vi "func_SendERR.vi"(6 "MoreINFO":string, 8 "ERR (String\\Errclust)":variant, 11 "YTESTER测试数据 in":T1) -> (3 "YTESTER测试数据 out":T1)   [LabVIEW 2017]
uses:
  YtCommon.lvlibp/yt`Step TestData.ctl
  YtCommon.lvlibp/yt`Step System Queue.ctl
  YtCommon.lvlibp
panel:
  # "This for Step vi"
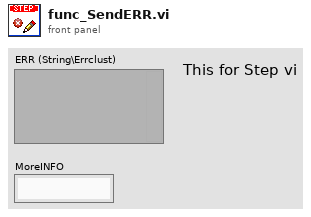
[diagram p1: front panel]
types:
  T1 = typedef "YtCommon.lvlibp/yt`Step TestData.ctl" = cluster{"Socket(From1)":i32, "SN":refnum<notifier>, "StopFlagRef":refnum<notifier>, "YT System Queue":refnum<queue>}
  T2 = typedef "YtCommon.lvlibp/yt`Step System Queue.ctl" = cluster{"Socket(From0)":i32, "Cmd":string, "Data":variant}
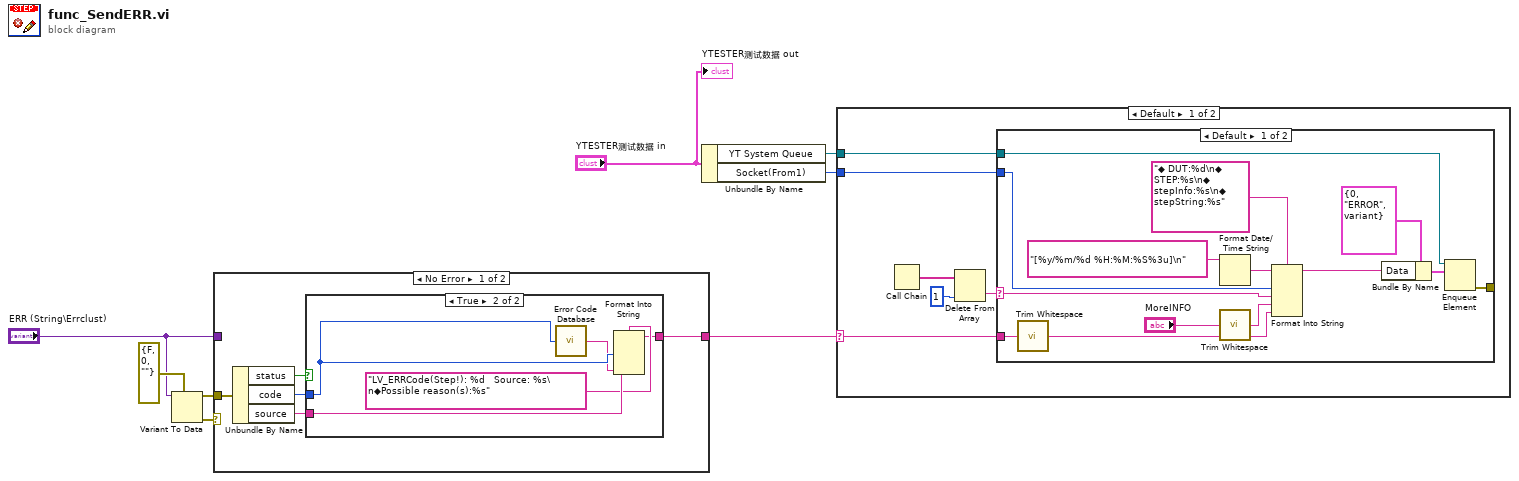
[diagram p0: block diagram]
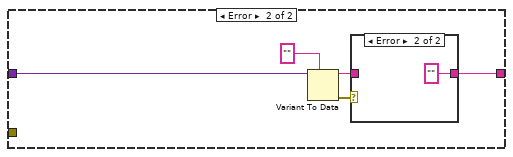
[diagram p5: hidden frame]
diagram:
  n1 = Variant To Data(type=errorcluster {"status"=FALSE, "code"=0, "source"=""} ("error constant"), Variant="ERR (String\\Errclust)") -> (data=w6:errorcluster, error out=w7:errorcluster)  [unwired: 1 in]
  n2 = case shown="No Error" w7 {
    tunnel: w6 -> [w13 _]
    tunnel: [w9 w20] -> w5
    tunnel: "ERR (String\\Errclust)" -> [_ w23]
    frame No Error {
      n3 = Unbundle By Name(w13) -> ("status"=w12:bool, "code"=w11:i32, "source"=w10:string)
      n4 = case shown="True" w12 {
        tunnel: w11 -> [_ w15]
        tunnel: w10 -> [_ w18]
        tunnel: [_ w16] -> w9
        frame False {
        }
        frame True {
          n5 = call <vilib>:"Error Code Database.vi"("Error Code"=w15) -> ("Error Text"=w14:string)
          n6 = Format Into String(format string="LV_ERRCode(Step!): %d   Source: %s\n◆Possible reason(s):%s", w15, w18, w14) -> (resulting string=w16:string)  [unwired: 2 in, 1 out]
        }
      }
    }
    frame Error {
      n7 = Variant To Data(type="", Variant=w23) -> (data=w19:string, error out=w21:errorcluster)  [unwired: 1 in]
      n8 = case shown="Error" w21 {
        tunnel: [w24 ""] -> w20
        tunnel: w19 -> [w24 _]
        frame No Error {
        }
        frame Error {
        }
      }
    }
  }
  n9 = Unbundle By Name("YTESTER测试数据 in") -> ("YT System Queue"=w1:refnum<queue>, "Socket(From1)"=w2:i32)
  n10 = case shown="Default" w5 {
    selector: w5 -> [w31 _]
    tunnel: w2 -> [w27 _]
    tunnel: w1 -> [w26 _]
    frame Default {
      n11 = Call Chain() -> (call chain=w30:string[])
      n12 = Delete From Array(array=w30, index=1) -> (deleted portion=w28:string)  [unwired: 1 in, 1 out]
      n13 = case shown="Default" w28 {
        selector: w28 -> [w44 _]
        tunnel: w31 -> [w43 _]
        tunnel: w27 -> [w34 _]
        tunnel: w26 -> [w35 _]
        tunnel: [w33 _] -> _
        frame Default {
          n14 = call <vilib>:"Trim Whitespace.vi"("string"=w43) -> ("trimmed string"=w38:string)  [unwired: 1 in]
          n15 = Format Date/Time String(time format string (%c)="[%y/%m/%d %H:%M:%S%3u]\n") -> (date/time string=w40:string)  [unwired: 2 in]
          n16 = call <vilib>:"Trim Whitespace.vi"("string"="MoreINFO") -> ("trimmed string"=w39:string)  [unwired: 1 in]
          n17 = Format Into String(format string="◆ DUT:%d\n◆ STEP:%s\n◆ stepInfo:%s\n◆ stepString:%s", initial string=w40, w34, w44, w39, w38) -> (resulting string=w32:string)  [unwired: 1 in, 1 out]
          n18 = Bundle By Name(cluster=T2 {"Socket(From0)"=0, "Cmd"="ERROR", "Data"=variant} ("element"), "Data"=w32) -> (w37:T2)
          n19 = Enqueue Element(queue=w35, element=w37) -> (error out=w33:errorcluster)  [unwired: 2 in, 2 out]
        }
        frame "" {
        }
      }
    }
    frame "" {
    }
  }
  "YTESTER测试数据 out" <- "YTESTER测试数据 in"
